vi "T7_Read_TEST.vi"() -> ()   [LabVIEW 2013]
uses:
  Serial Link Layer/NI_Modbus_Cleaned/NI Modbus121Clean.llb/MB Ethernet Master Query Read Input Registers (poly).vi
panel:
  out "TEST (UINT32) Value":u32
  in  "Num Registers":u16=2
  in  "Starting Address":u16=55100
  out "Results (binary)":u16[](array[numeric])
  in  "Remote IP Address":string="192.168.1.15"
  in  "Remote Port":u16=502
  in  "Stop":bool
  # "MB Ethernet Example Master.vi\n\nInstructions\n1.Use Kipling to find your devices IP address & modify the\n\"Remote IP Addres\"\n2. Run this VI to collect data for TEST or address 55100"
  # "TCP Parameters"
  # "Slave Read-only Registers"
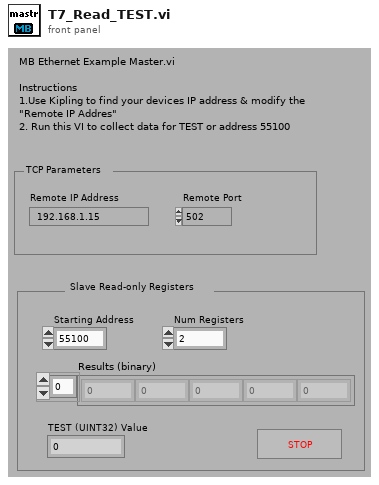
[diagram p1: front panel]
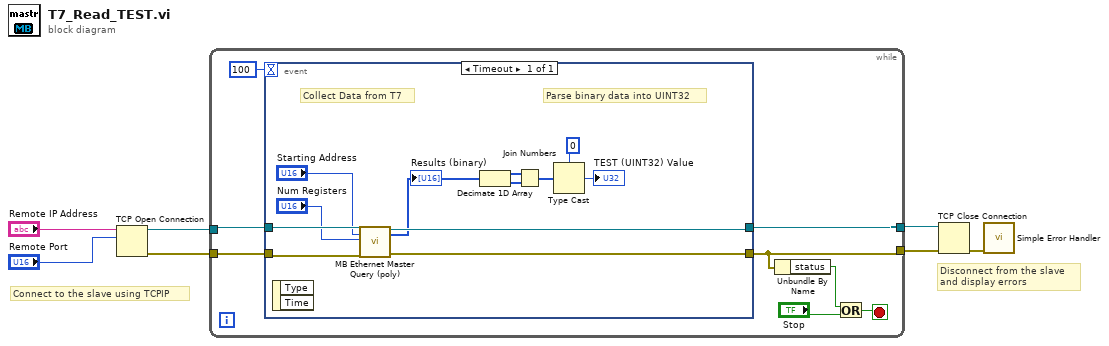
[diagram p0: block diagram]
diagram:
  # "Disconnect from the slave\nand display errors"
  # "Connect to the slave using TCPIP"
  n1 = TCP Open Connection(address="Remote IP Address", remote port or service name="Remote Port") -> (connection ID=w5:refnum<k5>, error out=w4:errorcluster)  [unwired: 3 in]
  n2 = while {
    tunnel: [w12] -> w2
    tunnel: w5 -> [w10]
    tunnel: w4 -> [w9]
    tunnel: [w8] -> w1
    stop <- w15 stop-if-true
    n3 = event shown="[0] Timeout" {
      selector: _ -> [_]
      dyn-events: _ -> [_]
      timeout: 100 -> [_]
      tunnel: [w22] -> w12
      tunnel: w10 -> [w27]
      tunnel: w9 -> [w25]
      tunnel: [w23] -> w8
      event Timeout {
        # "Parse binary data into UINT32"
        # "Collect Data from T7"
        n4 = event-data() -> ()  [unwired: 3 out]
        n5 = call-poly "MB Ethernet Master Query (poly).vi"("TCP Connection Refnum in"=w27, "Starting Address"="Starting Address", "Quantity"="Num Registers", "error in"=w25) -> ("TCP Connection Refnum (dup)"=w23:refnum<k5>, "Input Registers"=w21:u16[], "error out"=w22:errorcluster)  [unwired: 12 in, 1 out]
        "Results (binary)" <- w21
        n6 = Decimate 1D Array(w21) -> (w18:u16[], w17:u16[])
        n7 = Join Numbers(hi=w18, lo=w17) -> ((hi.lo)=w20:u32[])
        n8 = Type Cast(type=u32 0, x=w20) -> (*(type *) &x=→"TEST (UINT32) Value":u32)
      }
    }
    n9 = Unbundle By Name(w12) -> ("status"=w13:bool)
    n10 = Or(x=w13, y="Stop") -> (x .or. y?=w15:bool)
  }
  n11 = TCP Close Connection(connection ID=w1, error in (no error)=w2) -> (error out=w3:errorcluster)  [unwired: 2 out]
  n12 = call <vilib>:"Simple Error Handler.vi"("error in (no error)"=w3) -> ()  [unwired: 1 in, 8 out]
